vi "Part 2.vi"(11 "Input":string) -> (3 "Output":i64)   [LabVIEW 2020]
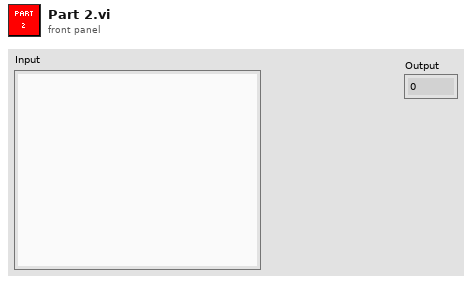
[diagram p1: front panel]
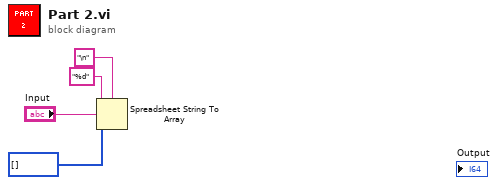
[diagram p0: block diagram]
diagram:
  n1 = Spreadsheet String To Array(delimiter (Tab)="\n", format string="%d", spreadsheet string="Input", array type (2D Dbl)=i32[] []) -> ()  [unwired: 1 out]
